vi "CoboltLaser_DriveCurrentSet.vi"(0 "ComPort":refnum<visa-resource-name>, 1 "LaserCurrent (mA)":dbl format="%.3g", 3 "CheckResponse":bool=TRUE, 7 "ErrorIn":errorcluster) -> (20 "ComPortOut":refnum<visa-resource-name>, 27 "ErrorOut":errorcluster)   [LabVIEW 2019]
doc: "Use this template to build a VI to use as a subVI."
panel:
  out "ResponseOK":bool
  out "Response":string
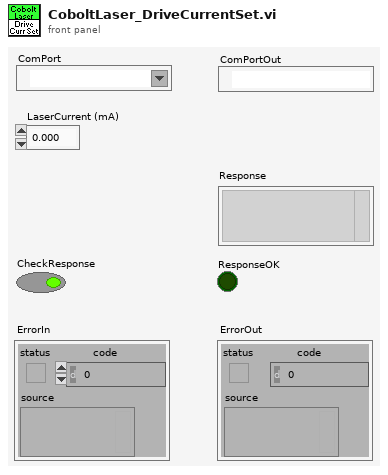
[diagram p1: front panel]
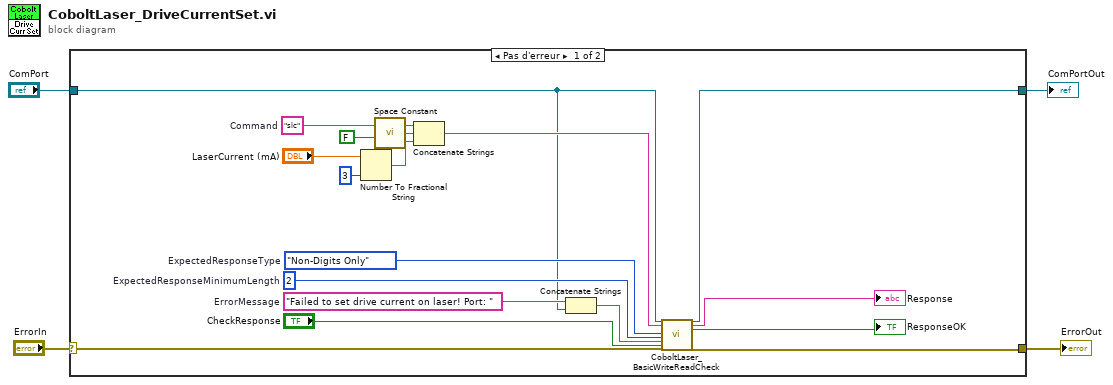
[diagram p0: block diagram]
diagram:
  n1 = case shown="Pas d'erreur" "ErrorIn" {
    selector: "ErrorIn" -> [w22 w24]
    tunnel: [w21 w24] -> w3
    tunnel: "ComPort" -> [w7 w23]
    tunnel: [w6 w23] -> w1
    frame No Error {
      w19 = 2  # ExpectedResponseMinimumLength
      w20 = enum16{"Any", "Digits Only", "Non-Digits Only"}."Non-Digits Only"  # ExpectedResponseType
      w15 = "Failed to set drive current on laser! Port: "  # ErrorMessage
      w13 = "slc"  # Command
      n2 = Number To Fractional String(use system decimal point (T)=FALSE, number="LaserCurrent (mA)", precision (6)=i16 3) -> (F-format string=w10:string)  [unwired: 1 in]
      n3 = call <vilib>:"Space Constant.vi"() -> ("String"=w12:string)
      n4 = Concatenate Strings(w13, w12, w10) -> (w9:string)
      n5 = Concatenate Strings(w15, w7) -> (w14:string)
      n6 = call <userlib>:"CoboltLaser_BasicWriteReadCheck.vi"("ComPort"=w7, "Command"=w9, "ExpectedResponseType"=w20, "ExpectedResponseMinimumLength"=w19, "ErrorMessage"=w14, "GenerateError"="CheckResponse", "error in (no error)"=w22) -> ("ComPortOut"=w6:refnum<visa-resource-name>, "Response"=→"Response":string, "ResponseOK"=→"ResponseOK":bool, "error out"=w21:errorcluster)  [unwired: 17 in]
    }
    frame Error {
    }
  }
  "ErrorOut" <- w3
  "ComPortOut" <- w1
